vi "Get Paths.vi"() -> (1 "Info Log":path, 2 "Config Log":path, 3 "Error Log":path)   [LabVIEW 2021, in "CIFLogs.lvlib"]
uses:
  CIFLogs.lvlib
  CIFConfigurationFile/CIF Configuration File.lvlib
  CIFConfigurationFile/typedef/Location Type.ctl
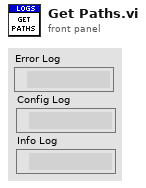
[diagram p1: front panel]
types:
  T1 = typedef "CIF Configuration File.lvlib/Location Type.ctl" = enum16{"Config File", "Manager", "Protos", "Plugins", "UI Plugins", "Logs"}
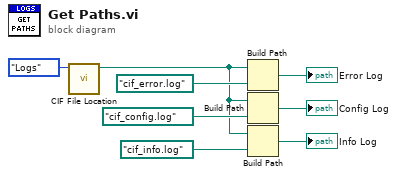
[diagram p0: block diagram]
diagram:
  n1 = call "CIF File Location.vi"("LocationType"=Location_Type."Logs") -> ("Location"=w4:path)  [unwired: 10 in]
  n2 = Build Path(base path=w4, name or relative path=path "cif_error.log" ("appended path")) -> (appended path=→"Error Log":path)
  n3 = Build Path(base path=w4, name or relative path=path "cif_config.log" ("appended path")) -> (appended path=→"Config Log":path)
  n4 = Build Path(base path=w4, name or relative path=path "cif_info.log" ("appended path")) -> (appended path=→"Info Log":path)
